vi "CleanUp.vi"(8 "error in (no error)":errorcluster, 11 "object in":refnum<class "CAN IO.lvclass">) -> (0 "error out":errorcluster, 3 "object out":refnum<class "CAN IO.lvclass">)   [LabVIEW 2013, in "CAN IO.lvclass"]
uses:
  CAN IO.lvclass
  CAN IO.lvclass/CAN IO.ctl
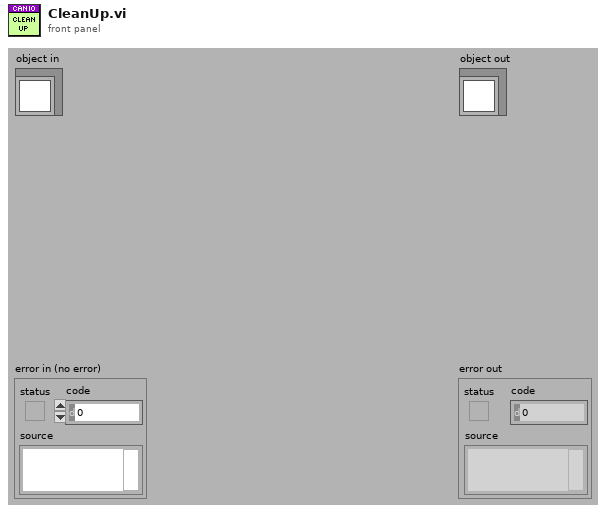
[diagram p1: front panel]
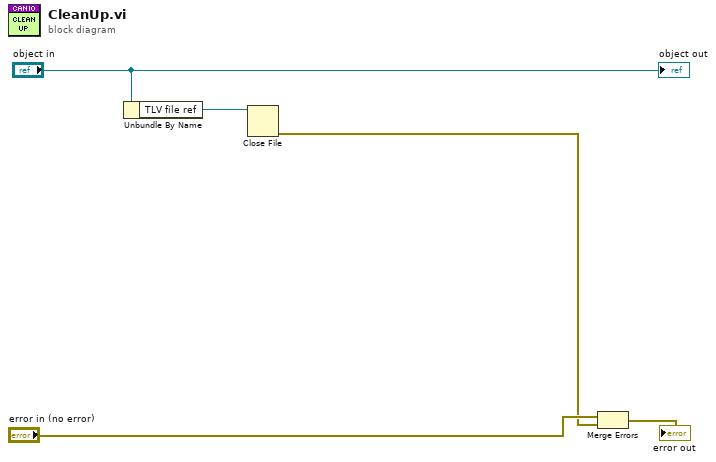
[diagram p0: block diagram]
diagram:
  n1 = Unbundle By Name("object in") -> ("TLV file ref"=w2:refnum<file>)
  n2 = Close File(refnum=w2) -> (error out=w1:errorcluster)  [unwired: 1 in, 1 out]
  n3 = Merge Errors("error in (no error)", w1) -> (→"error out":errorcluster)
  "object out" <- "object in"
